vi "Controls Tab.vi"(0 "Cube Intake Motor":dbl=1.0 min=0.0 max=10.0 step=1.0, 4 "Robot Lift Motor":dbl=1.0 min=0.0 max=10.0 step=1.0, 5 "Cube Lift Up Motor":dbl=1.0 min=0.0 max=10.0 step=1.0, 6 "Motor Controller Selection":string(combo)="Talon SRX", 7 "H-Wheel Motor Controller Selection":string(combo)="Talon SRX", 8 "Cube Lift Down Motor":dbl=1.0 min=0.0 max=10.0 step=1.0, 9 "X-AXIS":dbl=10.0 min=0.0 max=10.0 step=1.0, 10 "Y-AXIS":dbl=10.0 min=0.0 max=10.0 step=1.0, 11 "H-Wheel":dbl=10.0 min=0.0 max=10.0 step=1.0) -> ()   [LabVIEW 2017]
uses:
  <vilib>/Rock Robotics/Network Tables/NT Write Number.vi
  <vilib>/Rock Robotics/Network Tables/NT Write String.vi
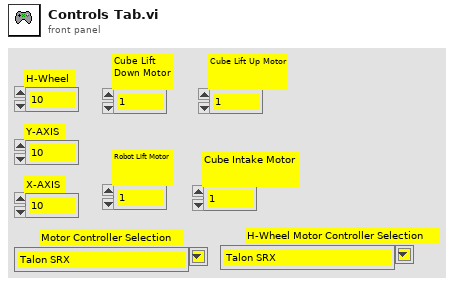
[diagram p1: front panel]
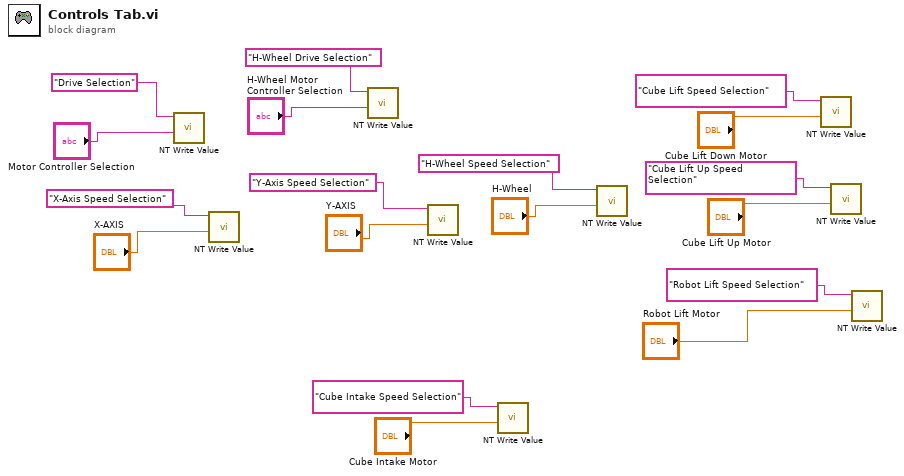
[diagram p0: block diagram]
diagram:
  n1 = call-poly <vilib>:"NT Write Value.vi"("String"="Motor Controller Selection", "Name"="Drive Selection") -> ()  [unwired: 9 in, 1 out]
  n2 = call-poly <vilib>:"NT Write Value.vi"("Numeric"="X-AXIS", "Name"="X-Axis Speed Selection") -> ()  [unwired: 9 in, 1 out]
  n3 = call-poly <vilib>:"NT Write Value.vi"("String"="H-Wheel Motor Controller Selection", "Name"="H-Wheel Drive Selection") -> ()  [unwired: 9 in, 1 out]
  n4 = call-poly <vilib>:"NT Write Value.vi"("Numeric"="Y-AXIS", "Name"="Y-Axis Speed Selection") -> ()  [unwired: 9 in, 1 out]
  n5 = call-poly <vilib>:"NT Write Value.vi"("Numeric"="Cube Intake Motor", "Name"="Cube Intake Speed Selection") -> ()  [unwired: 9 in, 1 out]
  n6 = call-poly <vilib>:"NT Write Value.vi"("Numeric"="H-Wheel", "Name"="H-Wheel Speed Selection") -> ()  [unwired: 9 in, 1 out]
  n7 = call-poly <vilib>:"NT Write Value.vi"("Numeric"="Cube Lift Down Motor", "Name"="Cube Lift Speed Selection") -> ()  [unwired: 9 in, 1 out]
  n8 = call-poly <vilib>:"NT Write Value.vi"("Numeric"="Cube Lift Up Motor", "Name"="Cube Lift Up Speed Selection") -> ()  [unwired: 9 in, 1 out]
  n9 = call-poly <vilib>:"NT Write Value.vi"("Numeric"="Robot Lift Motor", "Name"="Robot Lift Speed Selection") -> ()  [unwired: 9 in, 1 out]
